vi "Dashboard Main.vi"() -> ()   [LabVIEW 2012]
uses:
  <vilib>/event_ctls.llb/eventvkey.ctl
  <vilib>/Utility/config.llb/Read Key (String).vi
  <vilib>/Utility/config.llb/Read Key (I32).vi
  <vilib>/Utility/config.llb/Write Key (String).vi
  <vilib>/Utility/config.llb/Write Key (I32).vi
  <vilib>/Utility/config.llb/NI_LVConfig.lvlib
panel:
  in  "Camera Settings":T1={"Frate Rate"=30, "Compression"=30, "Size"=1} {"Frate Rate" scale=1.0..30.0; "Size" items=["640x480", "320x240", "160x120"]}
  out "Mode":T2(ring)=enum."Auto Disabled"
  in  "Viewer":T3(tab)
  out "Mbps":dbl format="%#.1g"
  in  "Enable":bool
  in  "DB Camera Config":bool
  out "Mbps":bool
  out "fps":dbl format="%#.1g"
  out "Image Error Message":string="Timeout in Camera Communications"
  out "Camera Image":T4(plugin-control)
  out "Camera Image 2":T4(plugin-control)
  out "fps 2":dbl format="%#.1g"
  out "Mbps 2":dbl format="%#.1g"
  in  "Enable 2":bool
  out "Camera IP 2":string
  out "Camera IP":string
  out "Buttons 1":cluster{"1":bool, "2":bool, "3":bool}
  out "Kinect 1":cluster{"X":dbl, "Y":dbl, "Z":dbl} {"X" scale=1.0..-1.0; "Y" scale=1.0..-1.0; "Z" scale=1.0..-1.0}
  out "Buttons 2":cluster{"1":bool, "2":bool, "3":bool}
  out "Kinect 2":cluster{"X":dbl, "Y":dbl, "Z":dbl} {"X" scale=1.0..-1.0; "Y" scale=1.0..-1.0; "Z" scale=1.0..-1.0}
  out "Version":string
  out "Skeleton Picture":picture
  out "Players":i8
  out "Robot IP":string
  out "Tree":string(tree)
  out "MotorSlide4":dbl(slide) scale=-1.0..1.0 scale format="%#_2e"
  out "MotorSlide3":dbl(slide) scale=-1.0..1.0 scale format="%#_2e"
  out "MotorSlide2":dbl(slide) scale=-1.0..1.0 scale format="%#_2e"
  in  "MotorName3":string="Front Left"
  in  "MotorName4":string="Front Right"
  in  "MotorName1":string="Rear Left"
  in  "MotorName2":string="Rear Right"
  out "MotorChart4":dbl(graph)
  out "MotorChart3":dbl(graph)
  out "MotorChart2":dbl(graph)
  out "MotorSlide1":dbl(slide) scale=-1.0..1.0 scale format="%#_2e"
  out "MotorChart1":dbl(graph)
  out "JS1 Z":dbl(slide) scale=-1.0..1.0 scale format="%#_2e"
  out "JS2 Z":dbl(slide) scale=-1.0..1.0 scale format="%#_2e"
  out "Joystick 1":cluster{"X":dbl, "Y":dbl}[](graph)
  out "Joystick 2":cluster{"X":dbl, "Y":dbl}[](graph)
  out "JS Buttons 1":T5
  out "JS Buttons 2":T5
  out "Battery Value":dbl(slide) scale=0.0..14.0 scale format="%#_2e"
  out "Battery":sgl(graph)
  in  "Dashboard Tab":enum32{"Operation", "Test", "Checklist"}(tab)
  in  "Checkbox 2":bool
  in  "Checkbox 1":bool
  in  "CIM 1 In":dbl(slide) scale=0.0..1.0
  in  "Slider":dbl(slide) scale=0.0..100.0 scale format="%#_3g"
  in  "On/Off":bool caption="Solenoid"
  in  "Test Name":u16(ring) items=["Select the test to run...", "Example Test", "-------------------------------", "List of tests is built in robot code.", "Replace with your own automated tests."]
  in  "Test Tree":string(tree)
  in  "Motor":cluster{"Value":dbl, "Enable":bool} {"Value" scale=-1.0..1.0 scale format="%#_3g"}
  out "Progress":T6 {"Test Progress" scale=0.0..100.0}
  in  "Rev/Fwd":cluster{"Forward":bool, "Reverse":bool}
  in  "Ring":u16(ring) items=["Auto", "Fixed indoor", "Fixed outdoor 1", "Fixed outdoor 2", "Fixed fluorescent 1", "Fixed fluorescent 2", "Hold current"]
  in  "Listbox":i32(listbox)
  # "Drive & Motors"
  # "Customize by placing controls and indicators here and name to match\nDashboard Variables on robot."
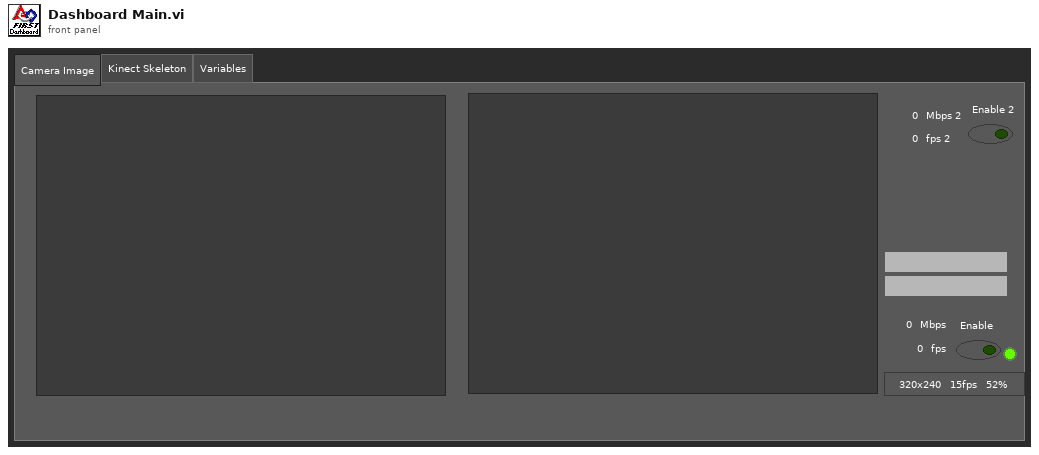
[diagram p1: front panel]
types:
  T1 = cluster{"Frate Rate":i32, "Compression":i32, "Size":u16}
  T2 = enum8{"Tele-Op Disabled", "Tele-Op Enabled", "Auto Disabled", "Auto Enabled", "Test Disabled", "Test Enabled", ""}
  T3 = enum32{"Camera Image", "Kinect Skeleton", "Variables"}
  T4 = typedef "IMAQ Image.ctl" = refnum<image>
  T5 = cluster{bool, bool, bool, bool, bool, bool, bool, bool, bool, bool, bool, bool}
  T6 = cluster{"Test Progress":u8, "Test Progress Text":string}
  T7 = typedef "Image Type" = u32
  T8 = typedef "LVBoundsTypeDef.ctl" = cluster{"Width":u32, "Height":u32}
  T9 = typedef "SkeletonTrackState.ctl" = enum32{"NotTracked", "PositionOnly", "Tracked"}
  T10 = cluster{"TrackingState":u8[], "Position":cluster{"x":sgl, "y":sgl, "z":sgl}, cluster{"x":sgl, "y":sgl, "z":sgl, sgl}[], "TrackState":T9}
  T11 = cluster{cluster{"ScaledToPercentRange":dbl, "ScaledToPercentRange":dbl, "ScaledToPercentRange":dbl}, cluster{bool, bool, bool}}[]
  T12 = cluster{cluster{"ScaledToPercentRange":dbl, "ScaledToPercentRange":dbl, "ScaledToPercentRange":dbl}, cluster{bool, bool, bool}}
  T13 = cluster{"ScaledToPercentRange":dbl, "ScaledToPercentRange":dbl, "ScaledToPercentRange":dbl}
  T14 = typedef "LVRectTypeDef.ctl" = cluster{"Left":i16, "Top":i16, "Right":i16, "Bottom":i16}
  T15 = cluster{"Competition mode":bool, "Robot Link":bool, "Autonomous":bool, "Enabled":bool, "E-Stop":bool, "Simulated":bool, "TestMode":bool, "Docked Window":bool}
  T16 = cluster{"Boolean Array[0]":bool, "Boolean Array[1]":bool, "Boolean Array[2]":bool, "Boolean Array[3]":bool, "Boolean Array[4]":bool, "Boolean Array[5]":bool, "Boolean Array[6]":bool, "Boolean Array[7]":bool, "Boolean Array[8]":bool, "Boolean Array[9]":bool, "Boolean Array[10]":bool, "Boolean Array[11]":bool}
  T17 = typedef "NI_LVConfig.lvlib/Config Data RefNum.ctl" = refnum<k1>
  T18 = typedef "eventvkey.ctl" = enum16{"ASCII", "Enter", "Return", "Shift", "Ctrl", "Alt", "Cmd", "Opt", "Caps", "NumLock", "Clear", "Break", "Up", "Down", "Left", "Right", "Insert", "Delete", "Home", "End", "PageUp", "PageDown", "Escape", "Help", "Pause", "ScrollLock", "F1", "F2", "F3", "F4", "F5", "F6", "F7", "F8", "F9", "F10", "F11", "F12", "F13", "F14", "F15", "F16", "F17", "F18", "F19", "F20", "F21", "F22", "F23", "F24", "Play", "VolumeUp", "VolumeDown", "Mute", "Two Byte Char"}
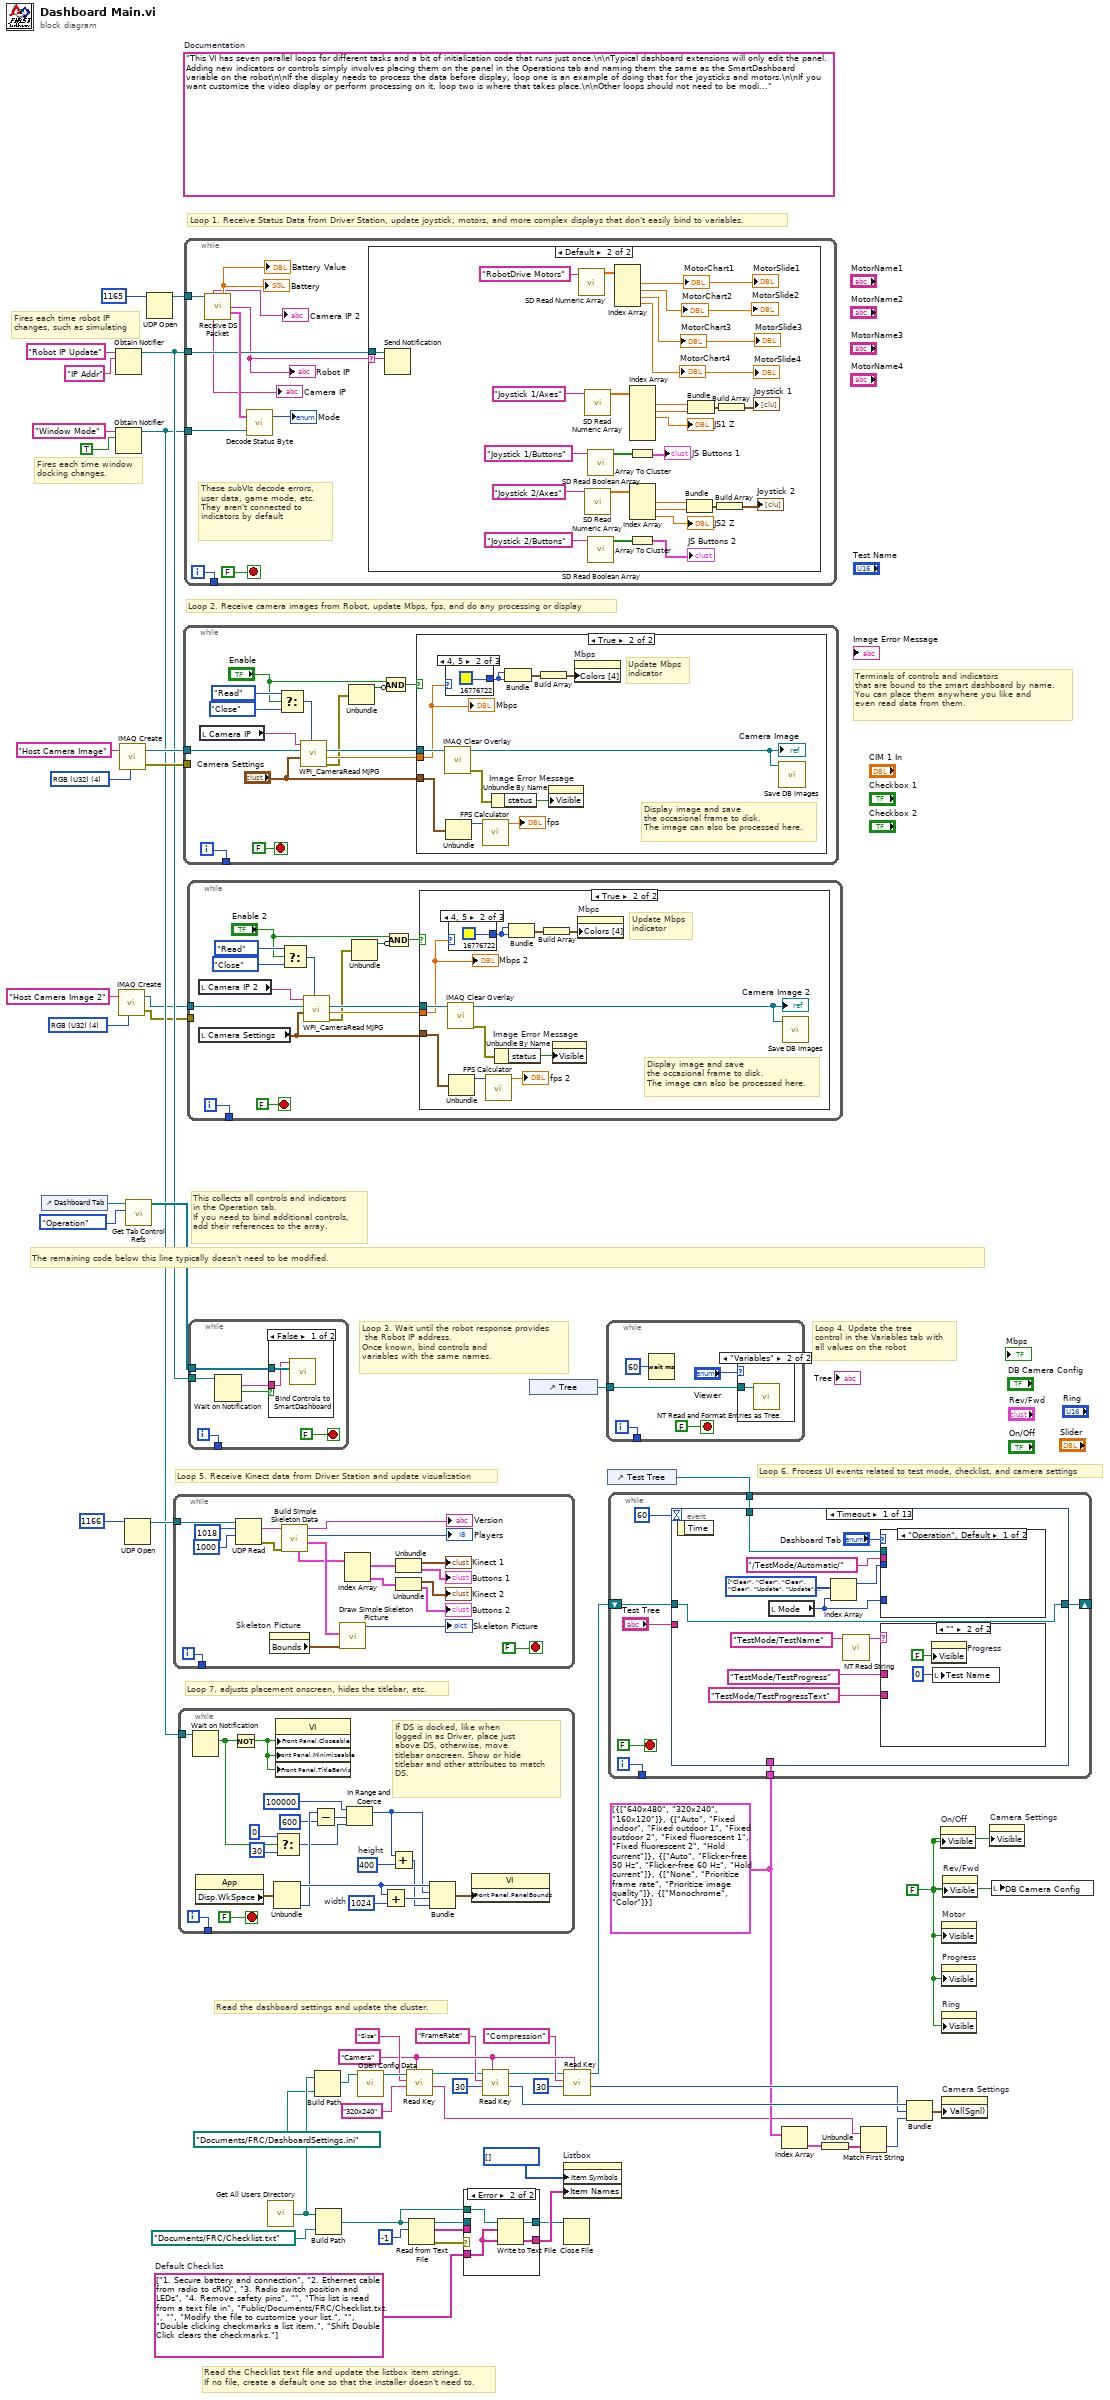
[diagram p0: block diagram]
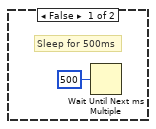
[diagram p2: hidden frame]
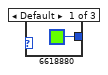
[diagram p3: hidden frame]
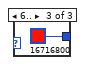
[diagram p4: hidden frame]
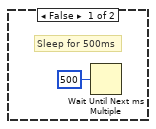
[diagram p6: hidden frame]
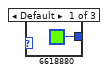
[diagram p7: hidden frame]
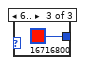
[diagram p8: hidden frame]
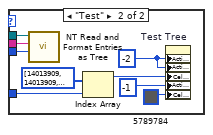
[diagram p10: hidden frame]
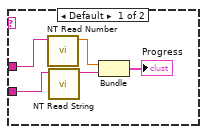
[diagram p11: hidden frame]
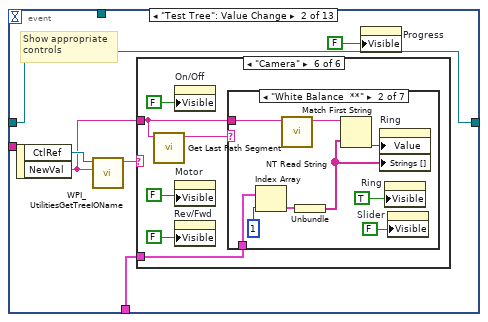
[diagram p12: hidden frame]
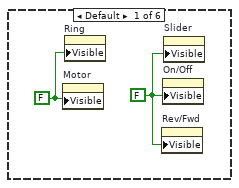
[diagram p13: hidden frame]
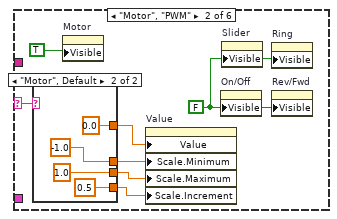
[diagram p14: hidden frame]
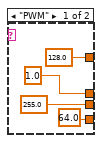
[diagram p15: hidden frame]
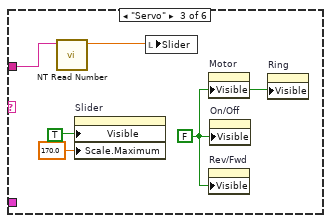
[diagram p16: hidden frame]
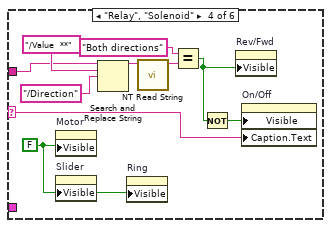
[diagram p17: hidden frame]
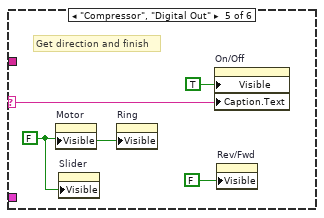
[diagram p18: hidden frame]
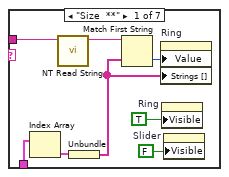
[diagram p19: hidden frame]
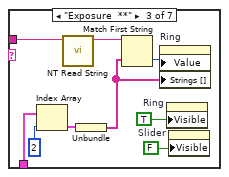
[diagram p20: hidden frame]
diagram:
  w3 = T7 4 items=["Grayscale (U8)", "Grayscale (I16)", "Grayscale (SGL)", "Complex (CSG)", "RGB (U32)", "HSL (U32)", "RGB (U64)"] ("Image Type")
  w25 = "Camera"
  w17 = cluster{string[]}[] [{["640x480", "320x240", "160x120"]}, {["Auto", "Fixed indoor", "Fixed outdoor 1", "Fixed outdoor 2", "Fixed fluorescent 1", "Fixed fluorescent 2", "Hold current"]}, {["Auto", "Flicker-free 50 Hz", "Flicker-free 60 Hz", "Hold current"]}, {["None", "Prioritize frame rate", "Prioritize image quality"]}, {["Monochrome", "Color"]}]
  w33 = string[] ["1. Secure battery and connection", "2. Ethernet cable from radio to cRIO", "3. Radio switch position and LEDs", "4. Remove safety pins", "", "This list is read from a text file in", "Public/Documents/FRC/Checklist.txt.", "", "Modify the file to customize your list.", "", "Double clicking checkmarks a list item.", "Shift Double Click clears the checkmarks."]  # Default Checklist
  w31 = FALSE ("Visible")
  (unwired) "This VI has seven parallel loops for different tasks and a bit of initialization code that runs just once.\n\nTypical dashboard extensions will only edit the panel. Adding new indicators or controls simply involves placing them on the panel in the Operations tab and naming them the same as the SmartDashboard variable on the robot\n\nIf the display needs to process the data before display, loop one is an example of doing that for the joysticks and motors.\n\nIf you want customize the video display or perform processing on it, loop two is where that takes place.\n\nOther loops should not need to be modified. They are pretty standard, and document the task they perform."  # Documentation
  w54 = T7 4 items=["Grayscale (U8)", "Grayscale (I16)", "Grayscale (SGL)", "Complex (CSG)", "RGB (U32)", "HSL (U32)", "RGB (U64)"] ("Image Type")
  # "Fires each time robot IP\nchanges, such as simulating"
  # "Fires each time window\ndocking changes."
  # "Read the Checklist text file and update the listbox item strings.\nIf no file, create a default one so that the installer doesn't need to."
  # "This collects all controls and indicators\nin the Operation tab.\nIf you need to bind additional controls,\nadd their references to the array."
  # "The remaining code below this line typically doesn't need to be modified."
  # "Loop 6. Process UI events related to test mode, checklist, and camera settings"
  # "Read the dashboard settings and update the cluster."
  # "Terminals of controls and indicators\nthat are bound to the smart dashboard by name.\nYou can place them anywhere you like and\neven read data from them."
  # "Loop 4. Update the tree\ncontrol in the Variables tab with\nall values on the robot"
  # "Loop 3. Wait until the robot response provides\n the Robot IP address.\nOnce known, bind controls and\nvariables with the same names."
  # "Loop 5. Receive Kinect data from Driver Station and update visualization"
  # "Loop 7. adjusts placement onscreen, hides the titlebar, etc."
  # "Loop 1. Receive Status Data from Driver Station, update joystick, motors, and more complex displays that don't easily bind to variables."
  # "Loop 2. Receive camera images from Robot, update Mbps, fps, and do any processing or display"
  n1 = control-ref of="Dashboard Tab"() -> (w47:refnum<vi>)
  n2 = Obtain Notifier(name (unnamed)="Robot IP Update", notification data type="IP Addr" ("name (unnamed)")) -> (notifier out=w44:refnum<notifier>)  [unwired: 2 in, 2 out]
  n3 = Obtain Notifier(name (unnamed)="Window Mode", notification data type=TRUE) -> (notifier out=w37:refnum<notifier>)  [unwired: 2 in, 2 out]
  n4 = call "IMAQ Create"("Image Name"="Host Camera Image 2", "Image Type"=w3) -> ("New Image"=w2:T4, "error out"=w1:errorcluster)  [unwired: 2 in, 1 out]
  n5 = call "IMAQ Create"("Image Name"="Host Camera Image", "Image Type"=w54) -> ("New Image"=w52:T4, "error out"=w51:errorcluster)  [unwired: 2 in, 1 out]
  n6 = UDP Open(11:u16 1166 ("port")) -> (port=w49:refnum<k16>)  [unwired: 2 in, 4 out]
  n7 = call <vilib>:"Get Tab Control Refs.vi"("Page Index"=enum32{"Operation", "Test"}."Operation" ("Dashboard Tab"), "TabControl in"=w47) -> ("ControlsOnPage"=w48:refnum<vi>[])  [unwired: 9 in]
  n8 = UDP Open(11:u16 1165 ("port")) -> (port=w55:refnum<k16>)  [unwired: 2 in, 4 out]
  n9 = while {
    tunnel: w49 -> [w73]
    tunnel: [w58] -> _
    i -> [w58]
    stop <- FALSE stop-if-true
    n10 = UDP Read(connection ID=w73, max size (548)=1018 ("bytes to read"), timeout ms (25000)=1000) -> (data out=w67:string, error out=w57:errorcluster)  [unwired: 1 in, 3 out]
    n11 = property on="Skeleton Picture" class="Pict"() -> ("Bounds"=w69:T8)  [unwired: 2 in, 2 out]
    n12 = call "Build Simple Skeleton Data.vi"("error in (no error)"=w57, "data in"=w67) -> ("Skeleton Data"=w68:T10, "NumPlayers"=→"Players":i8, "Version String"=→"Version":string, "Simple Joystick Info"=w65:T11)  [unwired: 5 in, 1 out]
    n13 = call "Draw Simple Skeleton Picture.vi"("Bounds"=w69, "Simple Skeleton"=w68) -> ("new picture out"=→"Skeleton Picture":picture)  [unwired: 9 in]
    n14 = Index Array(array=w65) -> (element #1=w64:T12, element #2=w63:T12)  [unwired: 2 in]
    n15 = Unbundle(w64) -> (→"Kinect 1":T13, →"Buttons 1":cluster{bool, bool, bool})
    n16 = Unbundle(w63) -> (→"Kinect 2":T13, →"Buttons 2":cluster{bool, bool, bool})
  }
  n17 = while {
    tunnel: w37 -> [w94]
    tunnel: [w92] -> _
    i -> [w92]
    stop <- FALSE stop-if-true
    w84 = 1024  # width
    w87 = 400  # height
    # "If DS is docked, like when\nlogged in as Driver, place just\nabove DS, otherwise, move\ntitlebar onscreen. Show or hide\ntitlebar and other attributes to match\nDS."
    n18 = Wait on Notification(notifier=w94) -> (notification=w79:bool)  [unwired: 3 in, 3 out]
    n19 = property class="App"() -> ("Disp.WkSpace"=w90:T14)  [unwired: 2 in, 2 out]
    n20 = Not(x=w79) -> (.not. x?=w93:bool)
    n21 = Unbundle(w90) -> ("Left"=w88:i16, "Bottom"=w85:i16)  [unwired: 2 out]
    n22 = Select(t=0, s=w79, f=30) -> (s? t:f=w78:i32)
    n23 = property class="VI"("Front Panel.Closeable"=w93, "Front Panel.Minimizeable"=w93, "Front Panel.TitleBarVis"=w93) -> ()  [unwired: 2 in, 2 out]
    n24 = Subtract(x=w85, y=600) -> (x-y=w82:i32)
    n25 = In Range and Coerce(upper limit=100000, x=w82, lower limit=w78) -> (coerced(x)=w76:i32)  [unwired: 1 out]
    n26 = Add(x=w88, y=w84) -> (x+y=w89:i32)
    n27 = Add(x=w76, y=w87) -> (x+y=w86:i32)
    n28 = Bundle("Left"=w88, w76, w89, w86) -> (w91:cluster{"Left":i16, i32, i32, i32})  [unwired: 1 out]
    n29 = property class="VI"("Front Panel.PanelBounds"=w91) -> ()  [unwired: 2 in, 2 out]
  }
  n30 = while {
    tunnel: w52 -> [w106]
    tunnel: w51 -> [_]
    tunnel: [w108] -> _
    i -> [w108]
    stop <- FALSE stop-if-true
    n31 = local read "Camera IP"() -> (w96:string)
    n32 = Select(t=enum16{"Read", "Reopen", "Close"}."Read" ("Operation"), s="Enable", f=enum16{"Read", "Reopen", "Close"}."Close" ("Operation")) -> (s? t:f=w101:enum16{"Read", "Reopen", "Close"})
    n33 = call <vilib>:"WPI_CameraRead MJPG.vi"("Operation"=w101, "Camera Settings"="Camera Settings", "Image"=w106, "address"=w96) -> ("error out"=w100:errorcluster, "Bandwidth (kbps)"=w104:dbl, "Image Out"=w105:T4)  [unwired: 5 in]
    n34 = Unbundle(w100) -> ("status"=w98:bool)  [unwired: 2 out]
    n35 = Compound Arithmetic op=AND("Enable", invert w98) -> (w97:bool)
    n36 = case shown="True" w97 {
      tunnel: "Camera Settings" -> [_ w112]
      tunnel: w105 -> [_ w115]
      tunnel: w104 -> [_ w114]
      frame False {
        # "Sleep for 500ms"
        n37 = Wait Until Next ms Multiple(millisecond multiple=u32 500) -> ()  [unwired: 1 out]
      }
      frame True {
        # "Display image and save\nthe occasional frame to disk.\nThe image can also be processed here."
        # "Update Mbps\nindicator"
        n38 = call "IMAQ Clear Overlay"("Image"=w115) -> ("error out"=w120:errorcluster, "Image Out"=w119:T4)  [unwired: 2 in, 7 out]
        "Camera Image" <- w119
        n39 = case shown="4, 5" w114 {
          tunnel: [u32 6618880 ("Color Box") u32 16776722 ("Color Box") u32 16716800 ("Color Box")] -> w116
          frame Default {
          }
          frame 4, 5 {
          }
          frame 6.. {
          }
        }
        n40 = Unbundle(w112) -> ("Frate Rate"=w111:i32)  [unwired: 2 out]
        n41 = call "FPS Calculator.vi"("Average Count"=w111) -> ("fps"=→"fps":dbl)  [unwired: 10 in]
        n42 = Unbundle By Name(w120) -> ("status"=w121:bool)
        n43 = Bundle("Color Box"=w116, "Color Box"=w116) -> (w118:cluster{"Color Box":u32, "Color Box":u32})  [unwired: 1 out]
        n44 = Build Array(w118) -> (w117:cluster{"Color Box":u32, "Color Box":u32}[])
        n45 = property on="Image Error Message" class="Str"("Visible"=w121) -> ()  [unwired: 2 in, 2 out]
        n46 = property on="Mbps" class="Bool (strict)"("Colors [4]"=w117) -> ()  [unwired: 2 in, 2 out]
        n47 = call "Save DB Images.vi"("Image"=w119) -> ()  [unwired: 2 in, 1 out]
        "Mbps" <- w114
      }
    }
  }
  n48 = while {
    tunnel: w55 -> [w133]
    tunnel: w44 -> [w128]
    tunnel: w37 -> [w131]
    tunnel: [w129] -> _
    i -> [w129]
    stop <- FALSE stop-if-true
    # "These subVIs decode errors, user data, game mode, etc.\nThey aren't connected to indicators by default"
    n49 = call "Receive DS Packet.vi"("Recv Socket"=w133) -> ("Camera IP Address 2"=→"Camera IP 2":string, "Battery"=→"Battery" →"Battery Value":sgl, "Robot IP Address"=w127:string, "Status"=w134:T15, "Camera IP Address"=→"Camera IP":string)  [unwired: 1 in, 9 out]
    "Robot IP" <- w127
    n50 = call "Decode Status Byte.vi"("Window Mode Notifier"=w131, "Status"=w134) -> ("Mode"=→"Mode":T2)  [unwired: 1 out]
    n51 = case shown="Default" w127 {
      selector: w127 -> [_ w136]
      tunnel: w128 -> [_ w137]
      frame "0.0.0.0" {
        # "Robot not responding, don't poll the variables"
      }
      frame Default {
        n52 = Send Notification(notification=w136, notifier=w137) -> ()  [unwired: 1 in, 2 out]
        n53 = call <vilib>:"SD Read Numeric Array.vi"("Name"="RobotDrive Motors") -> ("Numeric Array"=w160:dbl[])  [unwired: 8 in, 2 out]
        n54 = call <vilib>:"SD Read Numeric Array.vi"("Name"="Joystick 1/Axes") -> ("Numeric Array"=w153:dbl[])  [unwired: 8 in, 2 out]
        n55 = call <vilib>:"SD Read Numeric Array.vi"("Name"="Joystick 2/Axes") -> ("Numeric Array"=w147:dbl[])  [unwired: 8 in, 2 out]
        n56 = call <vilib>:"SD Read Boolean Array.vi"("Name"="Joystick 1/Buttons") -> ("Boolean Array"=w155:bool[])  [unwired: 8 in, 2 out]
        n57 = call <vilib>:"SD Read Boolean Array.vi"("Name"="Joystick 2/Buttons") -> ("Boolean Array"=w146:bool[])  [unwired: 8 in, 2 out]
        n58 = Index Array(array=w160) -> (element #1=→"MotorChart1" →"MotorSlide1":dbl, element #2=→"MotorSlide2" →"MotorChart2":dbl, element #3=→"MotorChart3" →"MotorSlide3":dbl, element #4=→"MotorChart4" →"MotorSlide4":dbl)  [unwired: 4 in]
        n59 = Array To Cluster(array=w155) -> (cluster=→"JS Buttons 1":T16)
        n60 = Array To Cluster(array=w146) -> (cluster=→"JS Buttons 2":T16)
        n61 = Index Array(array=w153) -> (element #1=w150:dbl, element #2=w151:dbl, element #3=→"JS1 Z":dbl)  [unwired: 6 in, 3 out]
        n62 = Index Array(array=w147) -> (element #1=w142:dbl, element #2=w141:dbl, element #3=→"JS2 Z":dbl)  [unwired: 3 in]
        n63 = Bundle("Numeric"=w142, "Numeric"=w141) -> (w143:cluster{"Numeric":dbl, "Numeric":dbl})  [unwired: 1 in]
        n64 = Bundle("Numeric"=w150, "Numeric"=w151) -> (w149:cluster{"Numeric":dbl, "Numeric":dbl})  [unwired: 1 in]
        n65 = Build Array(w143) -> (→"Joystick 2":cluster{"Numeric":dbl, "Numeric":dbl}[])
        n66 = Build Array(w149) -> (→"Joystick 1":cluster{"Numeric":dbl, "Numeric":dbl}[])
      }
    }
  }
  n67 = while {
    tunnel: w2 -> [w175]
    tunnel: [w176] -> _
    tunnel: w1 -> [_]
    i -> [w176]
    stop <- FALSE stop-if-true
    n68 = local read "Camera IP 2"() -> (w165:string)
    n69 = local read "Camera Settings"() -> (w164:T1)
    n70 = Select(t=enum16{"Read", "Reopen", "Close"}."Read" ("Operation"), s="Enable 2", f=enum16{"Read", "Reopen", "Close"}."Close" ("Operation")) -> (s? t:f=w170:enum16{"Read", "Reopen", "Close"})
    n71 = call <vilib>:"WPI_CameraRead MJPG.vi"("Operation"=w170, "Camera Settings"=w164, "Image"=w175, "address"=w165) -> ("error out"=w169:errorcluster, "Bandwidth (kbps)"=w173:dbl, "Image Out"=w174:T4)  [unwired: 5 in]
    n72 = Unbundle(w169) -> ("status"=w167:bool)  [unwired: 2 out]
    n73 = Compound Arithmetic op=AND("Enable 2", invert w167) -> (w166:bool)
    n74 = case shown="True" w166 {
      tunnel: w164 -> [_ w180]
      tunnel: w174 -> [_ w183]
      tunnel: w173 -> [_ w182]
      frame False {
        # "Sleep for 500ms"
        n75 = Wait Until Next ms Multiple(millisecond multiple=u32 500) -> ()  [unwired: 1 out]
      }
      frame True {
        # "Display image and save\nthe occasional frame to disk.\nThe image can also be processed here."
        # "Update Mbps\nindicator"
        n76 = call "IMAQ Clear Overlay"("Image"=w183) -> ("error out"=w188:errorcluster, "Image Out"=w187:T4)  [unwired: 2 in, 7 out]
        "Camera Image 2" <- w187
        n77 = case shown="4, 5" w182 {
          tunnel: [u32 6618880 ("Color Box") u32 16776722 ("Color Box") u32 16716800 ("Color Box")] -> w184
          frame Default {
          }
          frame 4, 5 {
          }
          frame 6.. {
          }
        }
        n78 = Unbundle(w180) -> ("Frate Rate"=w179:i32)  [unwired: 2 out]
        n79 = call "FPS Calculator.vi"("Average Count"=w179) -> ("fps"=→"fps 2":dbl)  [unwired: 10 in]
        n80 = Unbundle By Name(w188) -> ("status"=w189:bool)
        n81 = Bundle("Color Box"=w184, "Color Box"=w184) -> (w186:cluster{"Color Box":u32, "Color Box":u32})  [unwired: 1 out]
        n82 = Build Array(w186) -> (w185:cluster{"Color Box":u32, "Color Box":u32}[])
        n83 = property on="Image Error Message" class="Str"("Visible"=w189) -> ()  [unwired: 2 in, 2 out]
        n84 = property on="Mbps" class="Bool (strict)"("Colors [4]"=w185) -> ()  [unwired: 2 in, 2 out]
        n85 = call "Save DB Images.vi"("Image"=w187) -> ()  [unwired: 2 in, 1 out]
        "Mbps 2" <- w182
      }
    }
  }
  n86 = while {
    tunnel: w48 -> [w198]
    tunnel: w44 -> [w195]
    tunnel: [w193] -> _
    i -> [w193]
    stop <- FALSE stop-if-true
    n87 = Wait on Notification(notifier=w195) -> (notification=w194:string, timed out?=w196:bool)  [unwired: 3 in, 2 out]
    n88 = case shown="False" w196 {
      tunnel: w198 -> [w200 _]
      tunnel: w194 -> [w199 _]
      frame False {
        n89 = call <vilib>:"Bind Controls to SmartDashboard.vi"("Bound Control Refs"=w200, "Server IP Address"=w199) -> ()  [unwired: 10 in]
      }
      frame True {
      }
    }
  }
  n90 = call "Get All Users Directory.vi"() -> ("All User Path"=w30:path)
  n91 = Build Path(base path=w30, name or relative path=path "Documents/FRC/DashboardSettings.ini") -> (appended path=w29:path)
  n92 = Build Path(base path=w30, name or relative path=path "Documents/FRC/Checklist.txt") -> (appended path=w34:path)
  n93 = call <vilib>:"Open Config Data.vi"("configuration file path"=w29) -> ("refnum"=w28:T17)  [unwired: 8 in, 2 out]
  n94 = call-poly <vilib>:"Read Key.vi"("section"=w25, "default value"="320x240", "key"="Size", "refnum"=w28) -> ("value"=w15:string, "refnum out"=w10:T17)  [unwired: 2 in, 4 out]
  n95 = Read from Text File(file (use dialog)=w34, count=-1 ("timeout ms (25000)")) -> (refnum out=w12:refnum<file>, text=w35:string[], error out=w36:errorcluster)  [unwired: 2 in, 1 out]
  n96 = case shown="Error" w36 {
    tunnel: w35 -> [w202 _]
    tunnel: [w202 w204] -> w32
    tunnel: w33 -> [_ w204]
    tunnel: w34 -> [_ w205]
    tunnel: [w201 w203] -> w11
    tunnel: w12 -> [w201 _]
    frame No Error {
    }
    frame Error {
      n97 = Write to Text File(file (use dialog)=w205, text=w204) -> (refnum out=w203:refnum<file>)  [unwired: 2 in, 2 out]
    }
  }
  n98 = call-poly <vilib>:"Read Key.vi"("section"=w25, "default value"=30, "key"="FrameRate", "refnum"=w10) -> ("value"=w20:i32, "refnum out"=w9:T17)  [unwired: 1 in, 5 out]
  n99 = control-ref of="Tree"() -> (w6:refnum<vi>)
  n100 = property on="Listbox" class="LstBox (strict)"("Item Symbols"=i32[] [], "Item Names"=w32) -> ()  [unwired: 2 in, 2 out]
  n101 = Close File(refnum=w11) -> ()  [unwired: 1 in, 2 out]
  n102 = call-poly <vilib>:"Read Key.vi"("section"=w25, "default value"=30, "key"="Compression", "refnum"=w9) -> ("value"=w19:i32, "refnum out"=w7:T17)  [unwired: 1 in, 5 out]
  n103 = while {
    tunnel: [w207] -> _
    tunnel: w6 -> [w206]
    i -> [w207]
    stop <- FALSE stop-if-true
    n104 = Wait (ms)(milliseconds to wait=u32 60) -> ()  [unwired: 1 out]
    n105 = case shown="\"Variables\"" "Viewer" {
      tunnel: w206 -> [_ w211]
      frame Default {
      }
      frame "Variables" {
        n106 = call <vilib>:"NT Read and Format Entries as Tree.vi"("Tree Refnum"=w211) -> ()  [unwired: 9 in, 2 out]
      }
    }
  }
  n107 = control-ref of="Test Tree"() -> (w5:refnum<vi>)
  n108 = while {
    tunnel: w17 -> [w216]
    shift-right: [w215] -> _
    shift-left: w7 -> [w214]
    tunnel: [w213] -> _
    tunnel: w5 -> [w212]
    i -> [w213]
    stop <- FALSE stop-if-true
    n109 = event shown="[0] Timeout" {
      selector: _ -> [_ _ _ _ _ _ _ _ _ _ _ _ _]
      dyn-events: _ -> [_ _ _ _ _ _ _ _ _ _ _ _ _]
      timeout: u32 60 ("milliseconds to wait") -> [_ _ _ _ _ _ _ _ _ _ _ _ _]
      tunnel: w212 -> [w226 _ _ _ _ _ _ _ _ _ _ _ _]
      tunnel: "Test Tree" -> [_ _ _ _ _ _ _ _ w420 w428 w430 w434 w442]
      tunnel: w216 -> [_ w248 _ _ _ _ w384 w414 _ _ _ _ _]
      tunnel: [w220 w247 _ w350 w358 w370 w383 w407 w419 w426 w429 w433 w441] -> w215
      tunnel: w214 -> [w220 w247 _ w350 w358 w370 w382 w407 w419 w426 w429 w433 w441]
      event Timeout {
        w225 = enum16{"Update", "Clear"}[] [enum."Clear", enum."Clear", enum."Clear", enum."Clear", enum."Update", enum."Update", enum."Clear"] items=["Update", "Clear"]
        n110 = event-data() -> ()  [unwired: 1 in, 1 out]
        n111 = local read "Mode"() -> (w223:T2)
        n112 = Index Array(array=w225, index=w223) -> (element=w224:enum16{"Update", "Clear"})
        n113 = call <vilib>:"NT Read String.vi"("Name"="TestMode/TestName") -> ("String"=w229:string)  [unwired: 9 in, 1 out]
        n114 = case shown="\"Operation\", Default" "Dashboard Tab" {
          tunnel: w226 -> [_ w239]
          tunnel: "/TestMode/Automatic/" ("Name Pattern") -> [_ w238]
          tunnel: w224 -> [_ w237]
          tunnel: w223 -> [_ w235]
          frame "Operation", Default {
          }
          frame "Test" {
            w234 = -2 ("Active Item:Row Number")
            n115 = call <vilib>:"NT Read and Format Entries as Tree.vi"("Operation"=w237, "Name Pattern"=w238, "Tree Refnum"=w239) -> ()  [unwired: 7 in, 2 out]
            n116 = Index Array(array=u32[] [14013909, 14013909, 14013909, 14013909, 14013909, 16777215, 14013909], index=w235) -> (element=w233:u32)
            n117 = property on="Test Tree" class="Tree (strict)"("Active Item Row Number"=w234, "ActiveColNum"=w234, "CellBG"=w233, "Active Item Row Number"=-1 ("Active Item:Row Number"), "CellBG"=u32 5789784 ("Color Box")) -> ()  [unwired: 2 in, 2 out]
          }
        }
        n118 = case shown="\"\"" w229 {
          tunnel: "TestMode/TestProgress" ("Name") -> [w241 _]
          tunnel: "TestMode/TestProgressText" ("Name") -> [w240 _]
          frame Default {
            n119 = call <vilib>:"NT Read Number.vi"("Name"=w241) -> ("Numeric"=w242:dbl)  [unwired: 9 in, 1 out]
            n120 = call <vilib>:"NT Read String.vi"("Name"=w240) -> ("String"=w243:string)  [unwired: 9 in, 1 out]
            n121 = Bundle("Numeric"=w242, "String"=w243) -> (→"Progress":cluster{"Numeric":dbl, "String":string})  [unwired: 1 in]
          }
          frame "" {
            n122 = property on="Progress" class="Clust (strict)"("Visible"=FALSE) -> ()  [unwired: 2 in, 2 out]
            n123 = local write "Test Name"(u16 0) -> ()
          }
        }
      }
      event "Test Tree": Value Change {
        # "Show appropriate\ncontrols"
        n124 = event-data() -> ("CtlRef"=w251:refnum<vi>, "NewVal"=w249:string)  [unwired: 1 in]
        n125 = call <vilib>:"WPI_UtilitiesGetTreeIOName.vi"("NewVal"=w249, "TreeControl in"=w251) -> ("I/O Name"=w252:string)  [unwired: 9 in]
        n126 = case shown="\"Camera\"" w252 {
          selector: w252 -> [_ w259 _ w277 w286 _]
          tunnel: w249 -> [_ _ w274 w276 _ w293]
          tunnel: w248 -> [_ _ _ _ _ w292]
          frame Default {
            w254 = FALSE ("Visible")
            w253 = FALSE ("Visible")
            n127 = property on="Motor" class="Clust (strict)"("Visible"=w253) -> ()  [unwired: 2 in, 2 out]
            n128 = property on="Ring" class="Ring (strict)"("Visible"=w253) -> ()  [unwired: 2 in, 2 out]
            n129 = property on="Rev/Fwd" class="Clust (strict)"("Visible"=w254) -> ()  [unwired: 2 in, 2 out]
            n130 = property on="On/Off" class="Bool (strict)"("Visible"=w254) -> ()  [unwired: 2 in, 2 out]
            n131 = property on="Slider" class="Slide (strict)"("Visible"=w254) -> ()  [unwired: 2 in, 2 out]
          }
          frame "Motor", "PWM" {
            w260 = FALSE ("Visible")
            n132 = case shown="\"Motor\", Default" w259 {
              tunnel: [1.0 ("Value") -1.0 ("Value")] -> w258
              tunnel: [255.0 ("Value") 1.0 ("Value")] -> w257
              tunnel: [128.0 ("Value") 0.0 ("Value")] -> w256
              tunnel: [64.0 ("Value") 0.5 ("Value")] -> w255
              frame "PWM" {
              }
              frame "Motor", Default {
              }
            }
            n133 = property on="Motor" class="Clust (strict)"("Visible"=TRUE) -> ()  [unwired: 2 in, 2 out]
            n134 = property on="Value" class="Slide (strict)"("Value"=w256, "Scale.Minimum"=w258, "Scale.Maximum"=w257, "Scale.Increment"=w255) -> ()  [unwired: 2 in, 2 out]
            n135 = property on="On/Off" class="Bool (strict)"("Visible"=w260) -> ()  [unwired: 2 in, 2 out]
            n136 = property on="Slider" class="Slide (strict)"("Visible"=w260) -> ()  [unwired: 2 in, 2 out]
            n137 = property on="Ring" class="Ring (strict)"("Visible"=w260) -> ()  [unwired: 2 in, 2 out]
            n138 = property on="Rev/Fwd" class="Clust (strict)"("Visible"=w260) -> ()  [unwired: 2 in, 2 out]
          }
          frame "Servo" {
            w272 = FALSE ("Visible")
            n139 = call <vilib>:"NT Read Number.vi"("Name"=w274) -> ("Numeric"=w273:dbl)  [unwired: 9 in, 1 out]
            n140 = property on="Slider" class="Slide (strict)"("Visible"=TRUE, "Scale.Maximum"=170.0 ("Scale.Range:Maximum")) -> ()  [unwired: 2 in, 2 out]
            n141 = local write "Slider"(w273) -> ()
            n142 = property on="Motor" class="Clust (strict)"("Visible"=w272) -> ()  [unwired: 2 in, 2 out]
            n143 = property on="Rev/Fwd" class="Clust (strict)"("Visible"=w272) -> ()  [unwired: 2 in, 2 out]
            n144 = property on="On/Off" class="Bool (strict)"("Visible"=w272) -> ()  [unwired: 2 in, 2 out]
            n145 = property on="Ring" class="Ring (strict)"("Visible"=w272) -> ()  [unwired: 2 in, 2 out]
          }
          frame "Relay", "Solenoid" {
            w275 = FALSE ("Visible")
            n146 = property on="Motor" class="Clust (strict)"("Visible"=w275) -> ()  [unwired: 2 in, 2 out]
            n147 = property on="Slider" class="Slide (strict)"("Visible"=w275) -> ()  [unwired: 2 in, 2 out]
            n148 = Search and Replace String(input string=w276, search string="/Value  **", replace string="/Direction") -> (result string=w282:string)  [unwired: 5 in, 3 out]
            n149 = property on="Ring" class="Ring (strict)"("Visible"=w275) -> ()  [unwired: 2 in, 2 out]
            n150 = call <vilib>:"NT Read String.vi"("Name"=w282) -> ("String"=w280:string)  [unwired: 9 in, 1 out]
            n151 = Equal?(x="Both directions", y=w280) -> (x = y?=w278:bool)
            n152 = Not(x=w278) -> (.not. x?=w279:bool)
            n153 = property on="Rev/Fwd" class="Clust (strict)"("Visible"=w278) -> ()  [unwired: 2 in, 2 out]
            n154 = property on="On/Off" class="Bool (strict)"("Visible"=w279, "Caption.Text"=w277) -> ()  [unwired: 2 in, 2 out]
          }
          frame "Compressor", "Digital Out" {
            w285 = FALSE ("Visible")
            # "Get direction and finish"
            n155 = property on="Motor" class="Clust (strict)"("Visible"=w285) -> ()  [unwired: 2 in, 2 out]
            n156 = property on="Slider" class="Slide (strict)"("Visible"=w285) -> ()  [unwired: 2 in, 2 out]
            n157 = property on="Ring" class="Ring (strict)"("Visible"=w285) -> ()  [unwired: 2 in, 2 out]
            n158 = property on="On/Off" class="Bool (strict)"("Visible"=TRUE, "Caption.Text"=w286) -> ()  [unwired: 2 in, 2 out]
            n159 = property on="Rev/Fwd" class="Clust (strict)"("Visible"=FALSE) -> ()  [unwired: 2 in, 2 out]
          }
          frame "Camera" {
            n160 = call <vilib>:"Get Last Path Segment.vi"("String in"=w293) -> ("String out"=w294:string)  [unwired: 10 in]
            n161 = property on="On/Off" class="Bool (strict)"("Visible"=FALSE) -> ()  [unwired: 2 in, 2 out]
            n162 = property on="Motor" class="Clust (strict)"("Visible"=FALSE) -> ()  [unwired: 2 in, 2 out]
            n163 = property on="Rev/Fwd" class="Clust (strict)"("Visible"=FALSE) -> ()  [unwired: 2 in, 2 out]
            n164 = case shown="\"White Balance  **\"" w294 {
              tunnel: w293 -> [w300 w309 w318 w327 w336 _ w342]
              tunnel: w292 -> [w298 w306 w315 w324 w333 _ _]
              frame "Size  **" {
                n165 = Index Array(array=w298) -> (element=w297:cluster{string[]})  [unwired: 1 in]
                n166 = call <vilib>:"NT Read String.vi"("Name"=w300) -> ("String"=w299:string)  [unwired: 9 in, 1 out]
                n167 = Unbundle(w297) -> (w295:string[])
                n168 = Match First String(2:w295, 3:w299) -> (0:w296:i32)  [unwired: 1 out]
                n169 = property on="Ring" class="Ring (strict)"("Value"=w296, "Strings []"=w295) -> ()  [unwired: 2 in, 2 out]
                n170 = property on="Ring" class="Ring (strict)"("Visible"=TRUE) -> ()  [unwired: 2 in, 2 out]
                n171 = property on="Slider" class="Slide (strict)"("Visible"=FALSE) -> ()  [unwired: 2 in, 2 out]
              }
              frame "White Balance  **" {
                n172 = Index Array(array=w306, index=1) -> (element=w307:cluster{string[]})
                n173 = call <vilib>:"NT Read String.vi"("Name"=w309) -> ("String"=w308:string)  [unwired: 9 in, 1 out]
                n174 = Unbundle(w307) -> (w304:string[])
                n175 = Match First String(2:w304, 3:w308) -> (0:w303:i32)  [unwired: 1 out]
                n176 = property on="Ring" class="Ring (strict)"("Value"=w303, "Strings []"=w304) -> ()  [unwired: 2 in, 2 out]
                n177 = property on="Ring" class="Ring (strict)"("Visible"=TRUE) -> ()  [unwired: 2 in, 2 out]
                n178 = property on="Slider" class="Slide (strict)"("Visible"=FALSE) -> ()  [unwired: 2 in, 2 out]
              }
              frame "Exposure  **" {
                n179 = Index Array(array=w315, index=2) -> (element=w316:cluster{string[]})
                n180 = call <vilib>:"NT Read String.vi"("Name"=w318) -> ("String"=w317:string)  [unwired: 9 in, 1 out]
                n181 = Unbundle(w316) -> (w312:string[])
                n182 = Match First String(2:w312, 3:w317) -> (0:w313:i32)  [unwired: 1 out]
                n183 = property on="Ring" class="Ring (strict)"("Value"=w313, "Strings []"=w312) -> ()  [unwired: 2 in, 2 out]
                n184 = property on="Ring" class="Ring (strict)"("Visible"=TRUE) -> ()  [unwired: 2 in, 2 out]
                n185 = property on="Slider" class="Slide (strict)"("Visible"=FALSE) -> ()  [unwired: 2 in, 2 out]
              }
              frame "Exposure Priority  **" {
                n186 = Index Array(array=w324, index=3) -> (element=w325:cluster{string[]})
                n187 = call <vilib>:"NT Read String.vi"("Name"=w327) -> ("String"=w326:string)  [unwired: 9 in, 1 out]
                n188 = Unbundle(w325) -> (w321:string[])
                n189 = Match First String(2:w321, 3:w326) -> (0:w322:i32)  [unwired: 1 out]
                n190 = property on="Ring" class="Ring (strict)"("Value"=w322, "Strings []"=w321) -> ()  [unwired: 2 in, 2 out]
                n191 = property on="Ring" class="Ring (strict)"("Visible"=TRUE) -> ()  [unwired: 2 in, 2 out]
                n192 = property on="Slider" class="Slide (strict)"("Visible"=FALSE) -> ()  [unwired: 2 in, 2 out]
              }
              frame "Color Enable  **" {
                n193 = Index Array(array=w333, index=4) -> (element=w334:cluster{string[]})
                n194 = call <vilib>:"NT Read String.vi"("Name"=w336) -> ("String"=w335:string)  [unwired: 9 in, 1 out]
                n195 = Unbundle(w334) -> (w330:string[])
                n196 = Match First String(2:w330, 3:w335) -> (0:w331:i32)  [unwired: 1 out]
                n197 = property on="Ring" class="Ring (strict)"("Value"=w331, "Strings []"=w330) -> ()  [unwired: 2 in, 2 out]
                n198 = property on="Ring" class="Ring (strict)"("Visible"=TRUE) -> ()  [unwired: 2 in, 2 out]
                n199 = property on="Slider" class="Slide (strict)"("Visible"=FALSE) -> ()  [unwired: 2 in, 2 out]
              }
              frame Default {
                n200 = property on="Ring" class="Ring (strict)"("Visible"=FALSE) -> ()  [unwired: 2 in, 2 out]
                n201 = property on="Slider" class="Slide (strict)"("Visible"=FALSE) -> ()  [unwired: 2 in, 2 out]
              }
              frame "Brightness  **", "Color Level  **", "Compression  **", "FPS  **", "Sharpness  **" {
                n202 = call <vilib>:"NT Read Number.vi"("Name"=w342) -> ("Numeric"=w341:dbl)  [unwired: 9 in, 1 out]
                n203 = local write "Slider"(w341) -> ()
                n204 = property on="Slider" class="Slide (strict)"("Visible"=TRUE, "Scale.Maximum"=100.0 ("Scale.Range:Maximum")) -> ()  [unwired: 2 in, 2 out]
                n205 = property on="Ring" class="Ring (strict)"("Visible"=FALSE) -> ()  [unwired: 2 in, 2 out]
              }
            }
          }
        }
        n206 = property on="Progress" class="Clust (strict)"("Visible"=FALSE) -> ()  [unwired: 2 in, 2 out]
      }
      event "Test Name": Mouse Enter {
        # "Populate the ring with the list of tests"
        n207 = event-data() -> ()  [unwired: 1 in, 1 out]
        n208 = call <vilib>:"NT Read String Array.vi"("Name"="TestMode/TestList") -> ("String Array"=w349:string[])  [unwired: 9 in, 1 out]
        n209 = Build Array (concatenate)("Select the test to run...", w349) -> (w348:string[])
        n210 = property on="Test Name" class="Ring (strict)"("Strings []"=w348) -> ()  [unwired: 2 in, 2 out]
      }
      event "Test Name": Value Change {
        w351 = FALSE ("Visible")
        # "Tell the robot the test name to run"
        n211 = event-data() -> ("NewVal"=w355:u16)  [unwired: 1 in]
        n212 = property on="Test Name" class="Ring (strict)"() -> ("Strings []"=w356:string[])  [unwired: 2 in, 2 out]
        n213 = local write "Progress"(T6 {"Test Progress"=0, "Test Progress Text"=""} ("Progress")) -> ()
        n214 = Index Array(array=w356, index=w355) -> (element=w354:string)
        n215 = call <vilib>:"NT Write String.vi"("String"=w354, "Name"="TestMode/TestName") -> ()  [unwired: 9 in, 1 out]
        n216 = property on="Progress" class="Clust (strict)"("Visible"=TRUE) -> ()  [unwired: 2 in, 2 out]
        n217 = property on="Motor" class="Clust (strict)"("Visible"=w351) -> ()  [unwired: 2 in, 2 out]
        n218 = property on="Slider" class="Slide (strict)"("Visible"=w351) -> ()  [unwired: 2 in, 2 out]
        n219 = property on="On/Off" class="Bool (strict)"("Visible"=w351) -> ()  [unwired: 2 in, 2 out]
        n220 = property on="Rev/Fwd" class="Clust (strict)"("Visible"=w351) -> ()  [unwired: 2 in, 2 out]
        n221 = property on="Ring" class="Ring (strict)"("Visible"=w351) -> ()  [unwired: 2 in, 2 out]
      }
      event "Listbox": Double Click {
        n222 = event-data() -> ("PlatMods.Shift"=w359:bool, "Row"=w361:i32)  [unwired: 1 in]
        n223 = case shown="False" w359 {
          tunnel: w361 -> [w365 _]
          tunnel: 1 -> [w364 _]
          frame False {
            n224 = property on="Listbox" class="LstBox (strict)"() -> ("Item Symbols"=w363:i32[])  [unwired: 2 in, 2 out]
            n225 = Replace Array Subset(array=w363, new element=w364, index=w365) -> (w362:i32[])
            n226 = property on="Listbox" class="LstBox (strict)"("Item Symbols"=w362) -> ()  [unwired: 2 in, 2 out]
          }
          frame True {
            w366 = 0 ("Top Row")
            n227 = property on="Listbox" class="LstBox (strict)"() -> ("Number of Rows"=w368:u32)  [unwired: 2 in, 2 out]
            n228 = Initialize Array(0, w368) -> (w367:i32[])
            n229 = property on="Listbox" class="LstBox (strict)"("Top Row"=w366, "Value"=w366, "Item Symbols"=w367) -> ()  [unwired: 2 in, 2 out]
          }
        }
      }
      event "Listbox": Key Down {
        n230 = event-data() -> ("VKey"=w372:T18)  [unwired: 1 in]
        n231 = case shown="\"Left\", \"Right\"" w372 {
          selector: w372 -> [w377 _]
          tunnel: eventvkey."Left" ("VKey") -> [w375 _]
          frame "Left", "Right" {
            n232 = Equal?(x=w375, y=w377) -> (x = y?=w376:bool)
            n233 = Select(t=0, s=w376, f=1) -> (s? t:f=w378:i32)
            n234 = property on="Listbox" class="LstBox (strict)"() -> ("Item Symbols"=w381:i32[])  [unwired: 2 in, 2 out]
            n235 = Replace Array Subset(array=w381, new element=w378, index="Listbox") -> (w380:i32[])
            n236 = property on="Listbox" class="LstBox (strict)"("Item Symbols"=w380) -> ()  [unwired: 2 in, 2 out]
          }
          frame Default {
          }
        }
      }
      event "DB Camera Config": Value Change {
        n237 = event-data() -> ("NewVal"=w385:bool)  [unwired: 1 in]
        n238 = case shown="False" w385 {
          tunnel: w384 -> [w394 _]
          tunnel: [w387 w405] -> w383
          tunnel: w382 -> [w386 w405]
          frame False {
            w401 = "Camera"
            w404 = FALSE ("Visible")
            n239 = local read "Camera Settings"() -> (w393:T1)
            n240 = Index Array(array=w394) -> (element=w397:cluster{string[]})  [unwired: 1 in]
            n241 = Unbundle(w393) -> ("Frate Rate"=w392:i32, "Compression"=w391:i32, "Size"=w395:u16)
            n242 = Unbundle(w397) -> (w396:string[])
            n243 = Index Array(array=w396, index=w395) -> (element=w390:string)
            n244 = call-poly <vilib>:"Write Key.vi"("section"=w401, "value"=w390, "key"="Size", "refnum"=w386) -> ("refnum out"=w403:T17)  [unwired: 2 in, 5 out]
            n245 = call-poly <vilib>:"Write Key.vi"("section"=w401, "value"=w392, "key"="FrameRate", "refnum"=w403) -> ("refnum out"=w402:T17)  [unwired: 1 in, 6 out]
            n246 = property on="Camera Settings" class="Clust (strict)"("Visible"=w404) -> ()  [unwired: 2 in, 2 out]
            n247 = local write "DB Camera Config"(w404) -> ()
            n248 = call-poly <vilib>:"Write Key.vi"("section"=w401, "value"=w391, "key"="Compression", "refnum"=w402) -> ("refnum out"=w388:T17)  [unwired: 1 in, 6 out]
            n249 = call <vilib>:"Close Config Data.vi"("refnum"=w388) -> ("file path"=w389:path)  [unwired: 2 in, 8 out]
            n250 = call <vilib>:"Open Config Data.vi"("configuration file path"=w389) -> ("refnum"=w387:T17)  [unwired: 8 in, 2 out]
          }
          frame True {
            n251 = property on="Camera Settings" class="Clust (strict)"("Visible"=TRUE) -> ()  [unwired: 2 in, 2 out]
          }
        }
      }
      event "Camera Settings": Value Change {
        n252 = event-data() -> ("NewVal"=w418:T1)  [unwired: 1 in]
        n253 = Index Array(array=w414) -> (element=w413:cluster{string[]})  [unwired: 1 in]
        n254 = Unbundle(w418) -> ("Frate Rate"=w409:i32, "Compression"=w408:i32, "Size"=w411:u16)
        n255 = Unbundle(w413) -> (w412:string[])
        n256 = Index Array(array=w412, index=w411) -> (element=w410:string)
        n257 = Format Into String(format string="%s   %dfps   %d%%", w410, w409, w408) -> (resulting string=w415:string)  [unwired: 2 in, 1 out]
        n258 = Build Array(w415) -> (w416:string[])
        n259 = property on="DB Camera Config" class="Bool (strict)"("Strings [4]"=w416) -> ()  [unwired: 2 in, 2 out]
      }
      event "Motor.Enable": Value Change {
        n260 = event-data() -> ("NewVal"=w424:bool)  [unwired: 1 in]
        n261 = Unbundle("Motor") -> ("Value"=w423:dbl)  [unwired: 1 out]
        n262 = Select(t=w423, s=w424, f=0.0) -> (s? t:f=w421:dbl)
        n263 = call <vilib>:"NT Write Number.vi"("Numeric"=w421, "Name"=w420) -> ()  [unwired: 9 in, 1 out]
      }
      event "Slider": Value Change {
        n264 = event-data() -> ("NewVal"=w427:dbl)  [unwired: 1 in]
        n265 = call <vilib>:"NT Write Number.vi"("Numeric"=w427, "Name"=w428) -> ()  [unwired: 9 in, 1 out]
      }
      event "On/Off": Value Change {
        n266 = event-data() -> ("NewVal"=w432:bool)  [unwired: 1 in]
        n267 = Boolean To (0,1)(Boolean=w432) -> (0, 1=w431:i16)
        n268 = call <vilib>:"NT Write Number.vi"("Numeric"=w431, "Name"=w430) -> ()  [unwired: 9 in, 1 out]
      }
      event "Rev/Fwd": Value Change {
        n269 = event-data() -> ("NewVal.Forward"=w440:bool, "NewVal.Reverse"=w439:bool)  [unwired: 1 in]
        n270 = Boolean To (0,1)(Boolean=w440) -> (0, 1=w436:i16)
        n271 = Boolean To (0,1)(Boolean=w439) -> (0, 1=w438:i16)
        n272 = Negate(x=w438) -> (-x=w437:i16)
        n273 = Add(x=w436, y=w437) -> (x+y=w435:i16)
        n274 = call <vilib>:"NT Write Number.vi"("Numeric"=w435, "Name"=w434) -> ()  [unwired: 9 in, 1 out]
      }
      event "Ring": Value Change {
        n275 = event-data() -> ("NewVal"=w444:u16)  [unwired: 1 in]
        n276 = property on="Ring" class="Ring (strict)"() -> ("Strings []"=w445:string[])  [unwired: 2 in, 2 out]
        n277 = Index Array(array=w445, index=w444) -> (element=w443:string)
        n278 = call <vilib>:"NT Write String.vi"("String"=w443, "Name"=w442) -> ()  [unwired: 9 in, 1 out]
      }
    }
  }
  n279 = Index Array(array=w17) -> (element=w18:cluster{string[]})  [unwired: 1 in]
  n280 = Unbundle(w18) -> (w16:string[])
  n281 = Match First String(2:w16, 3:w15) -> (0:w14:i32)  [unwired: 1 out]
  n282 = Bundle("value"=w20, "value"=w19, "index"=w14) -> (w8:cluster{"value":i32, "value":i32, "index":i32})  [unwired: 1 out]
  n283 = property on="On/Off" class="Bool (strict)"("Visible"=w31) -> ()  [unwired: 2 in, 2 out]
  n284 = property on="Motor" class="Clust (strict)"("Visible"=w31) -> ()  [unwired: 2 in, 2 out]
  n285 = property on="Progress" class="Clust (strict)"("Visible"=w31) -> ()  [unwired: 2 in, 2 out]
  n286 = property on="Ring" class="Ring (strict)"("Visible"=w31) -> ()  [unwired: 2 in, 2 out]
  n287 = property on="Camera Settings" class="Clust (strict)"("Val(Sgnl)"=w8) -> ()  [unwired: 2 in, 2 out]
  n288 = property on="Rev/Fwd" class="Clust (strict)"("Visible"=w31) -> ()  [unwired: 2 in, 2 out]
  n289 = property on="Camera Settings" class="Clust (strict)"("Visible"=w31) -> ()  [unwired: 2 in, 2 out]
  n290 = local write "DB Camera Config"(w31) -> ()
